vi "Acquire.vi"(8 "error in (no error)":errorcluster caption="错误输入（无错误）", 9 "Analog Data Queue":refnum<queue> caption="模拟数据队列", 10 "Angle Data Queue":refnum<queue> caption="角度数据队列", 11 "Hardware Resources in":T1={"电压读取设置"={"DAQmx Channel"="", "Max Input"=0.0, "Min Input"=0.0, "Sample Rate"=0.0, "Sample Number"=0, "DAQmx Task"="", "device in"=""}, "角度传感器设置"={"counter"="Dev1/ctr0", "units"=10146, "分辨率"=0, "初始角度"=0.0, "DecodingType"=10092, "A相端口"="/Dev1/PFI8", "B相端口"="/Dev1/PFI8", "task in"=""}} caption="硬件资源输入" {"角度传感器设置"."DecodingType" items=["X1"=10090, "X2"=10091, "X4"=10092, "Two Pulse Counting"=10313]; "角度传感器设置"."units" items=["Degrees"=10146, "Radians"=10273, "Ticks"=10304, "From Custom Scale"=10065]}) -> (0 "error out":errorcluster caption="错误输出", 3 "Hardware Resources out":T1={"电压读取设置"={"DAQmx Channel"="", "Max Input"=0.0, "Min Input"=0.0, "Sample Rate"=0.0, "Sample Number"=0, "DAQmx Task"="", "device in"=""}, "角度传感器设置"={"counter"="Dev1/ctr0", "units"=10146, "分辨率"=0, "初始角度"=0.0, "DecodingType"=10092, "A相端口"="/Dev1/PFI8", "B相端口"="/Dev1/PFI8", "task in"=""}} caption="硬件资源输出" {"角度传感器设置"."DecodingType" items=["X1"=10090, "X2"=10091, "X4"=10092, "Two Pulse Counting"=10313]; "角度传感器设置"."units" items=["Degrees"=10146, "Radians"=10273, "Ticks"=10304, "From Custom Scale"=10065]})   [LabVIEW 2015, in "Acquisition.lvlib"]
doc: "执行采集。替换程序框图的内容，添加对采集硬件的调用。"
uses:
  Acquisition.lvlib
  Hardware Configuration.ctl
  <vilib>/DAQmx/read.llb/DAQmx Read (Counter DBL 1Chan 1Samp).vi
  <vilib>/DAQmx/read.llb/DAQmx Read (Analog 2D DBL NChan NSamp).vi
  <vilib>/DAQmx/miscellaneous.llb/DAQmx Fill In Error Info.vi
  <resource>/objmgr/daqmx.rc
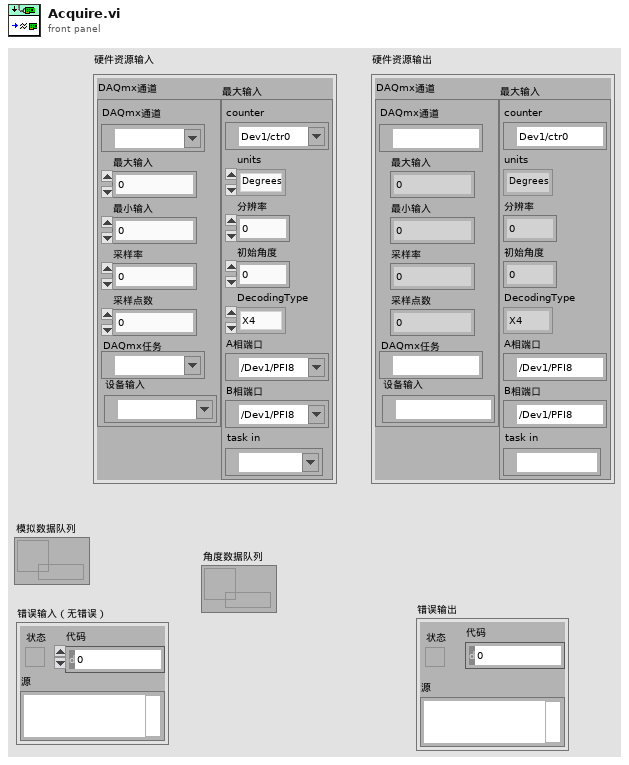
[diagram p1: front panel]
types:
  T1 = typedef "Acquisition.lvlib/Hardware Configuration.ctl" = cluster{"电压读取设置":cluster{"DAQmx Channel":tag, "Max Input":dbl, "Min Input":dbl, "Sample Rate":dbl, "Sample Number":i32, "DAQmx Task":refnum<k21>, "device in":tag}, "角度传感器设置":cluster{"counter":tag, "units":i32, "分辨率":i32, "初始角度":dbl, "DecodingType":i32, "A相端口":tag, "B相端口":tag, "task in":refnum<k21>}}
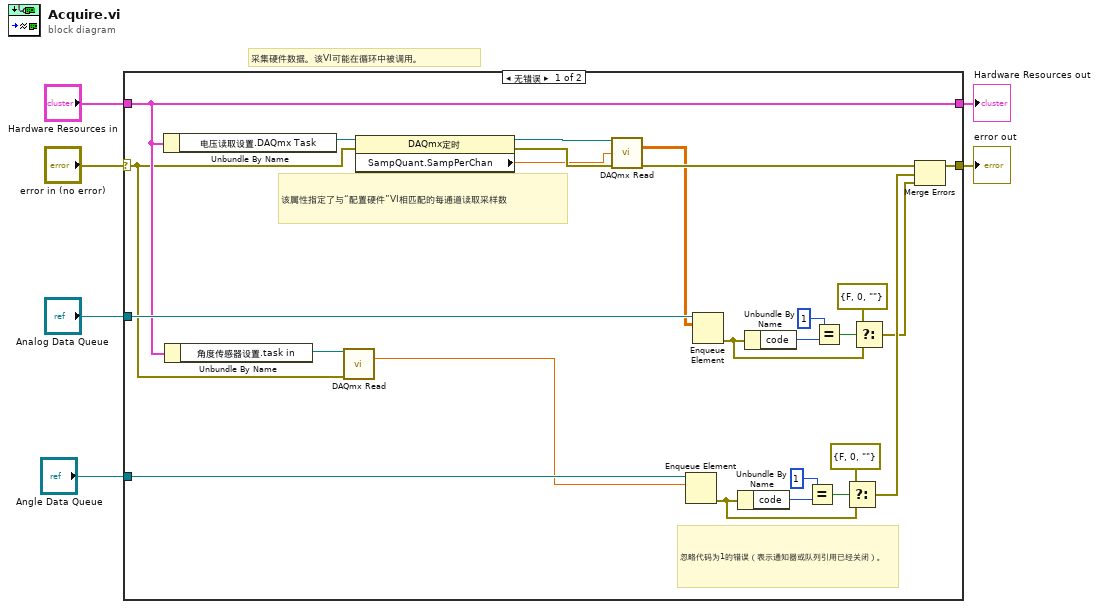
[diagram p0: block diagram]
diagram:
  # "采集硬件数据。该VI可能在循环中被调用。"
  n1 = case shown="无错误" "error in (no error)" {
    selector: "error in (no error)" -> [w9 w32]
    tunnel: [w31 w32] -> w5
    tunnel: "Hardware Resources in" -> [w11 w33]
    tunnel: [w11 w33] -> w3
    tunnel: "Analog Data Queue" -> [w18 _]
    tunnel: "Angle Data Queue" -> [w8 _]
    frame No Error {
      # "该属性指定了与“配置硬件”VI相匹配的每通道读取采样数"
      # "忽略代码为1的错误（表示通知器或队列引用已经关闭）。"
      n2 = Unbundle By Name(w11) -> ("电压读取设置.DAQmx Task"=w16:refnum<k21>)
      n3 = Unbundle By Name(w11) -> ("角度传感器设置.task in"=w10:refnum<k21>)
      n4 = call-poly <vilib>:"DAQmx Read.vi"("task/channels in"=w10, "error in"=w9) -> ("data"=w7:dbl)  [unwired: 11 in, 2 out]
      n5 = property class="DAQmx定时"(reference=w16, error in=w9) -> (reference out=w15:refnum<k21>, error out=w14:errorcluster, "SampQuant.SampPerChan"=w13:dbl)
      n6 = call-poly <vilib>:"DAQmx Read.vi"("task/channels in"=w15, "number of samples per channel"=w13, "error in"=w14) -> ("data"=w12:dbl[][], "error out"=w17:errorcluster)  [unwired: 10 in, 1 out]
      n7 = Enqueue Element(queue=w8, element=w7) -> (error out=w27:errorcluster)  [unwired: 2 in, 2 out]
      n8 = Enqueue Element(queue=w18, element=w12) -> (error out=w23:errorcluster)  [unwired: 2 in, 2 out]
      n9 = Unbundle By Name(w27) -> ("code"=w30:i32)
      n10 = Unbundle By Name(w23) -> ("code"=w20:i32)
      n11 = Equal?(x=1, y=w30) -> (x = y?=w28:bool)
      n12 = Equal?(x=1, y=w20) -> (x = y?=w22:bool)
      n13 = Select(t=errorcluster {"status"=FALSE, "code"=0, "source"=""} ("error constant"), s=w28, f=w27) -> (s? t:f=w26:errorcluster)
      n14 = Select(t=errorcluster {"status"=FALSE, "code"=0, "source"=""} ("error constant"), s=w22, f=w23) -> (s? t:f=w19:errorcluster)
      n15 = Merge Errors(w17, w26, w19) -> (w31:errorcluster)
    }
    frame Error {
    }
  }
  "Hardware Resources out" <- w3
  "error out" <- w5
